vi "RunExe-Send Target Ready.vi"(0 "instance":u16, 7 "Timeout (s)":dbl=1.0 format="%#_13g", 11 "error in (no error)":errorcluster) -> (15 "error out":errorcluster)   [LabVIEW 2020]
doc: "We use a \"launcher\" VI with splash screen to start the main executable. This is not simply a matter of aesthetics; some exe's take a few seconds to become visible and a few seconds longer to become functional during which time it appears that nothing is happening. In contrast, the splash screen appears immediately.\n\nProblem: how do we know when the main exe is ready and the launcher can be terminated? Ideally, the launcher should determine that on its own and the main exe should have no knowledge of the launcher. In practice, I don't find a reliable way to detect that. \n\nRejected solutions: the launcher could be part of the main VI, but that functionality doesn't really belong there. The launcher could load and run the main VI (in a single exe), but that the loading of the main VI from an exe is messy. Also, the main exe should stand on its own.\n\nSolution: we'll have the main exe broadcast one time over a socket that it is ready. It should not be an error if no one is listening for the broadcast.\n\nThis VI is used by the main exe to broadcast its readiness."
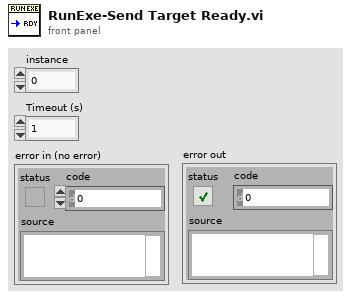
[diagram p1: front panel]
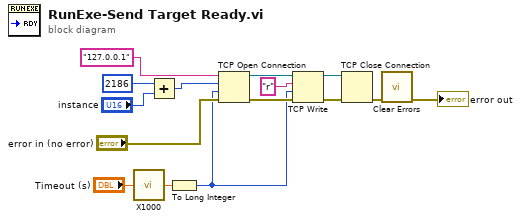
[diagram p0: block diagram]
diagram:
  n1 = call "X1000.vi"("X"="Timeout (s)") -> ("X/1000"=w11:dbl)
  n2 = Add(x=u16 2186 ("port"), y="instance") -> (x+y=w2:u16)
  n3 = To Long Integer(number=w11) -> (32bit integer=w6:i32)
  n4 = TCP Open Connection(address="127.0.0.1" ("name"), remote port or service name=w2, timeout ms (60000)=w6, error in (no error)="error in (no error)") -> (connection ID=w14:refnum<k5>, error out=w13:errorcluster)  [unwired: 1 in]
  n5 = TCP Write(connection ID=w14, data in="r", error in (no error)=w13, 9:w6) -> (connection ID out=w9:refnum<k5>, error out=w10:errorcluster)  [unwired: 1 out]
  n6 = TCP Close Connection(connection ID=w9, error in (no error)=w10) -> (error out=w8:errorcluster)  [unwired: 1 in, 1 out]
  n7 = call <vilib>:"Clear Errors.vi"("error in (no error)"=w8) -> ("error out"=→"error out":errorcluster)  [unwired: 5 in, 1 out]
